vi "list all functions.vi"(11 "user module configuration in":refnum<class "test 4 configuration.lvclass">) -> (2 "functions":string[](array[string]), 3 "user module configuration out":refnum<class "test 4 configuration.lvclass">)   [LabVIEW 2013]
uses:
  Users/blueuser/Documents/LabVIEW Data/test 4/module/configuration/test 4 configuration.lvclass
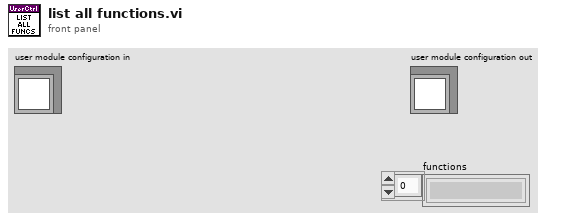
[diagram p1: front panel]
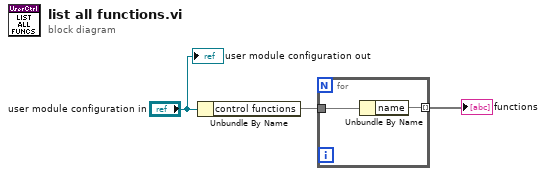
[diagram p0: block diagram]
diagram:
  n1 = Unbundle By Name("user module configuration in") -> ("control functions"=w2)
  n2 = for {
    tunnel: w2 -> [w5]
    tunnel: [w4] -> w1 mode=indexing
    n3 = Unbundle By Name(w5) -> ("name"=w4)
  }
  "functions" <- w1
  "user module configuration out" <- "user module configuration in"
